vi "niScope Fetch Binary 16.vi"(7 "timeout":dbl=5.0 format="%.2f", 8 "error in":errorcluster, 9 "numSamples":i32=-1, 10 "channels":string="0", 11 "instrument handle":refnum<k15>) -> (0 "error out":errorcluster, 1 "wfm":i16[](array[numeric]), 2 "wfm info":T1 {"reserved2" format="%.2f"; "reserved1" format="%.2f"; "offset" format="%^.3e"; "gain" format="%^.3e"; "xIncrement" format="%^.3e"; "relativeInitialX" format="%^.3e"; "absoluteInitialX" format="%^.3e"}, 3 "instrument handle out":refnum<k15>)   [LabVIEW 2011]
doc: "Retrieves data from a single channel and record. Returns a one-dimensional array of binary 16-bit values."
uses:
  niScope_32.dll
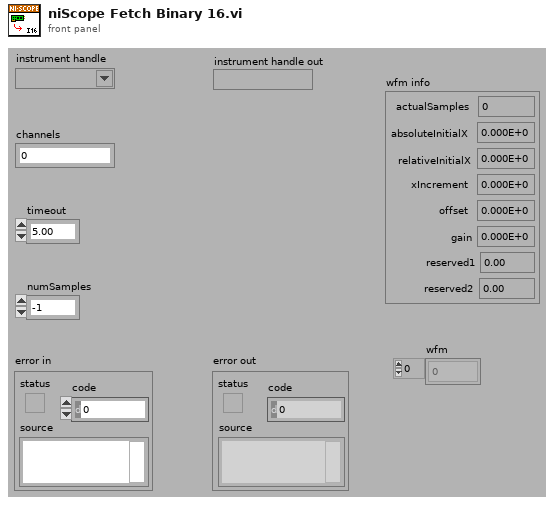
[diagram p1: front panel]
types:
  T1 = cluster{"actualSamples":i32, "absoluteInitialX":dbl, "relativeInitialX":dbl, "xIncrement":dbl, "offset":dbl, "gain":dbl, "reserved1":dbl, "reserved2":dbl}
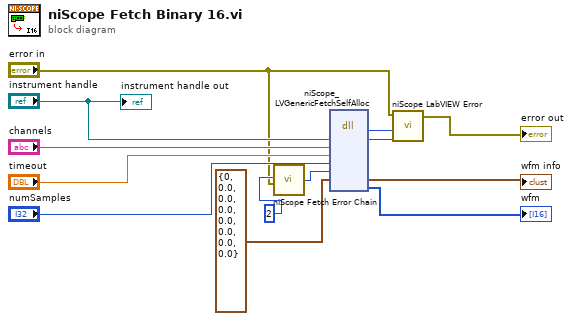
[diagram p0: block diagram]
diagram:
  n1 = call <instrlib>:"niScope Fetch Error Chain.vi"("dataType in"=2 ("dataType"), "error in"="error in") -> ("dataType"=w2:i32)  [unwired: 13 in]
  n2 = dll-call lib="niScope_*.*" fn="niScope_LVGenericFetchSelfAlloc"("instrument handle"="instrument handle", "channelList"="channels", "timeout"="timeout", "numSamples"="numSamples", "dataType"=w2, "wfmInfo"=T1 {"actualSamples"=0, "absoluteInitialX"=0.0, "relativeInitialX"=0.0, "xIncrement"=0.0, "offset"=0.0, "gain"=0.0, "reserved1"=0.0, "reserved2"=0.0}) -> ("status"=w4:i32, "instrument handle"=w3:u32, "wfmInfo"=→"wfm info":T1, "wfm"=→"wfm":i16[])  [unwired: 8 in, 2 out]
  n3 = call <instrlib>:"niScope LabVIEW Error.vi"("instrument handle"=w3, "niScope error code (0)"=w4, "error in (no error)"="error in") -> ("error out"=→"error out":errorcluster)  [unwired: 2 in]
  "instrument handle out" <- "instrument handle"
